vi "My Singleton Module teardown.vi"(8 "error in":errorcluster) -> (0 "error out":errorcluster)   [LabVIEW 2023]
doc: "_____\nCreated using DQMH Event Scripter 6.1.0.128."
uses:
  Libraries/My Singleton Module/My Singleton Module.lvlib
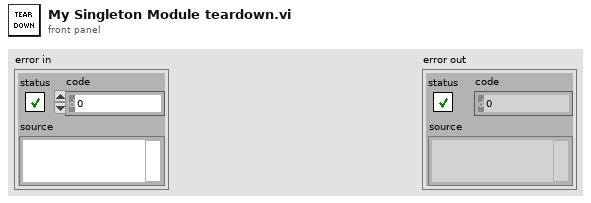
[diagram p1: front panel]
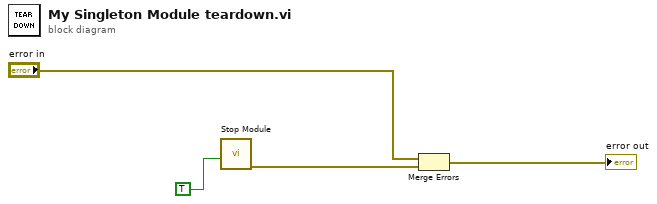
[diagram p0: block diagram]
diagram:
  n1 = call "Stop Module.vi"("Wait for Module to Stop? (F)"=TRUE) -> ("error out"=w4:errorcluster)  [unwired: 10 in]
  n2 = Merge Errors("error in", w4) -> (→"error out":errorcluster)
